vi "Reconfig.vi"(8 "error in (no error)":errorcluster, 11 "Agilent DSO-X 3032A in":refnum<class "Agilent DSO-X 3032A.lvclass">) -> (0 "error out":errorcluster, 3 "Agilent DSO-X 3032A out":refnum<class "Agilent DSO-X 3032A.lvclass">)   [LabVIEW 2014]
uses:
  Agilent DSO-X 3032A.lvclass
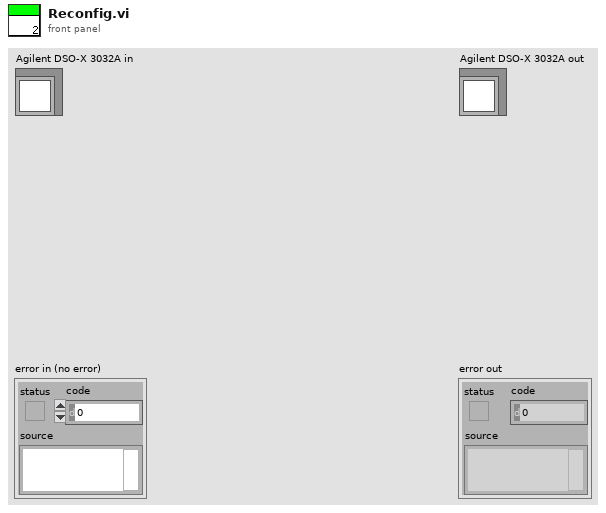
[diagram p1: front panel]
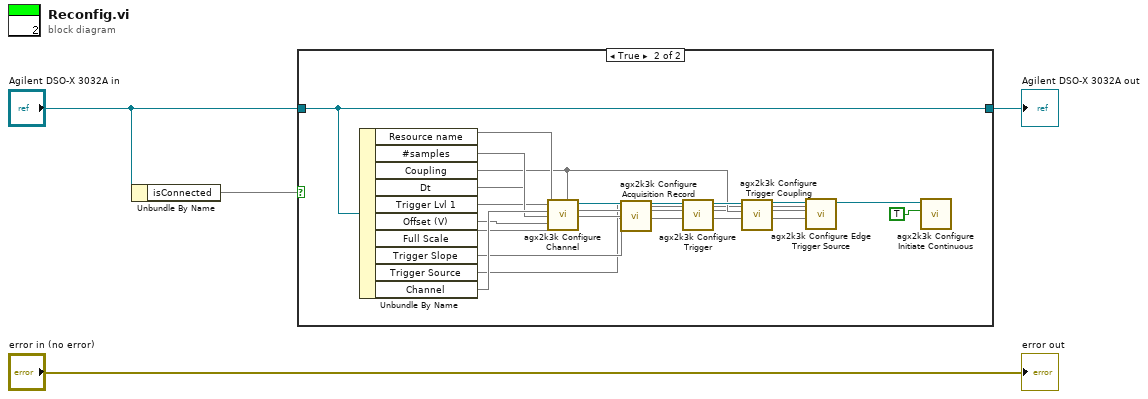
[diagram p0: block diagram]
diagram:
  n1 = Unbundle By Name("Agilent DSO-X 3032A in") -> ("isConnected"=w1)
  n2 = case shown="True" w1 {
    tunnel: [w5 w16] -> w4
    tunnel: "Agilent DSO-X 3032A in" -> [w5 w16]
    frame False {
    }
    frame True {
      n3 = Unbundle By Name(w16) -> ("Resource name"=w12, "#samples"=w14, "Coupling"=w9, "Dt"=w13, "Trigger Lvl 1"=w6, "Offset (V)"=w11, "Full Scale"=w10, "Trigger Slope"=w8, "Trigger Source"=w7, "Channel"=w15)
      n4 = call <instrlib>:"agx2k3k Configure Channel.vi"("vertical offset (0.0)"=w11, "vertical coupling (DC)"=w9, "vertical range (100.0e-3)"=w10, "channel name (\"CHAN1\")"=w15, "instrument handle"=w12) -> ("instrument handle out"=w17:refnum<k15>)  [unwired: 3 in, 3 out]
      n5 = call <instrlib>:"agx2k3k Configure Acquisition Record.vi"("instrument handle"=w17, "time per record (1E-3)"=w13, "min record length (1000)"=w14) -> ("instrument handle out"=w22:refnum<k15>)  [unwired: 2 in, 10 out]
      n6 = call <instrlib>:"agx2k3k Configure Trigger.vi"("instrument handle"=w22) -> ("instrument handle out"=w21:refnum<k15>)  [unwired: 3 in, 7 out]
      n7 = call <instrlib>:"agx2k3k Configure Trigger Coupling.vi"("trigger coupling (DC)"=w9, "instrument handle"=w21) -> ("instrument handle out"=w20:refnum<k15>)  [unwired: 1 in, 8 out]
      n8 = call <instrlib>:"agx2k3k Configure Edge Trigger Source.vi"("trigger slope (Positive)"=w8, "trigger level (0.0)"=w6, "trigger source (\"CHAN1\")"=w7, "instrument handle"=w20) -> ("instrument handle out"=w18:refnum<k15>)  [unwired: 1 in, 6 out]
      n9 = call <instrlib>:"agx2k3k Configure Initiate Continuous.vi"("continuous acquisition (False)"=TRUE, "instrument handle"=w18) -> ()  [unwired: 1 in, 9 out]
    }
  }
  "Agilent DSO-X 3032A out" <- w4
  "error out" <- "error in (no error)"
